vi "Open BD.vi"(8 "error in":errorcluster, 9 "Open BD":bool, 10 "Selected VIs":string[](array[string]), 11 "Application in":refnum<vi>) -> (0 "error out":errorcluster)   [LabVIEW 2013, in "LVTM.lvlib"]
uses:
  LVTM.lvlib
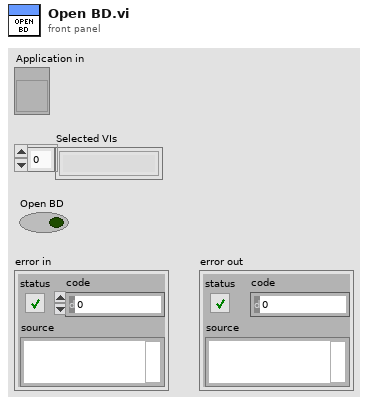
[diagram p1: front panel]
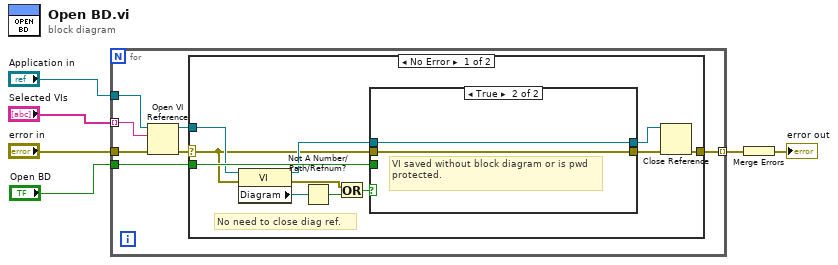
[diagram p0: block diagram]
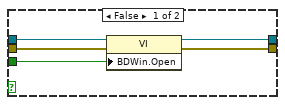
[diagram p2: hidden frame]
diagram:
  n1 = for {
    tunnel: [w13] -> w1 mode=indexing
    tunnel: "error in" -> [w12]
    tunnel: "Selected VIs" -> [w11] mode=indexing
    tunnel: "Application in" -> [w10]
    tunnel: "Open BD" -> [w9]
    n2 = Open VI Reference(application reference (local)=w10, vi path=w11, error in (no error)=w12) -> (vi reference=w8:refnum<vi>, error out=w7:errorcluster)  [unwired: 3 out]
    n3 = case shown="No Error" w7 {
      selector: w7 -> [w14 _]
      tunnel: [w24 _] -> w13
      tunnel: w9 -> [w21 _]
      tunnel: w8 -> [w20 _]
      frame No Error {
        # "No need to close diag ref."
        n4 = property class="VI"(reference=w20, error in=w14) -> (reference out=w19:refnum<vi>, error out=w16:errorcluster, "Diagram"=w18:refnum<vi>)
        n5 = Not A Number/Path/Refnum?(number/path/refnum=w18) -> (NaN/Path/Refnum?=w17:bool)
        n6 = Or(x=w16, y=w17) -> (x .or. y?=w15:bool)
        n7 = case shown="True" w15 {
          tunnel: [w29 w31] -> w23
          tunnel: [w28 w30] -> w22
          tunnel: w21 -> [w27 _]
          tunnel: w14 -> [w26 w30]
          tunnel: w19 -> [w25 w31]
          frame False {
            n8 = property class="VI"(reference=w25, error in=w26, "BDWin.Open"=w27) -> (reference out=w29:refnum<vi>, error out=w28:errorcluster)
          }
          frame True {
            # "VI saved without block diagram or is pwd protected."
          }
        }
        n9 = Close Reference(reference=w23, error in (no error)=w22) -> (error out=w24:errorcluster)
      }
      frame Error {
        # "This VI is no longer in the memory"
      }
    }
  }
  n10 = Merge Errors(w1) -> (→"error out":errorcluster)
